vi "灰度化 (子VI).vi"(8 "错误输入（无错误）":errorcluster, 11 "引用句柄输入":T1) -> (0 "错误输出":errorcluster, 2 "图像差分":T1(plugin-control), 3 "引用句柄输出":T1)   [LabVIEW 2012]
uses:
  <vilib>/vision/Image Controls.llb/IMAQ Image.ctl
  <vilib>/vision/NI_Vision_Development_Module.lvlib
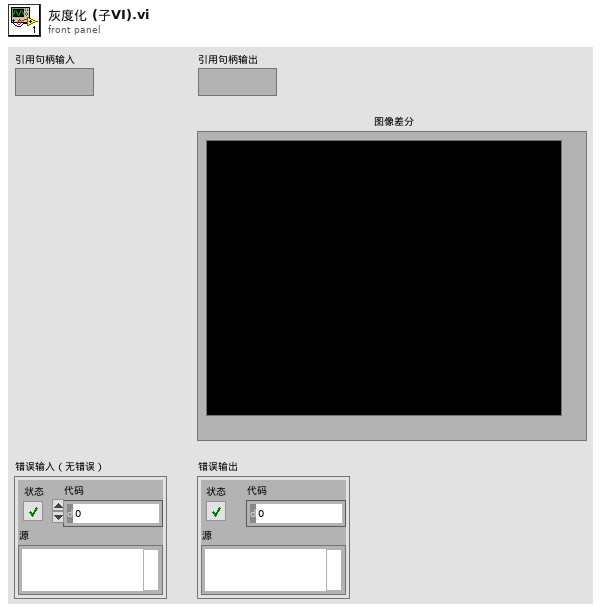
[diagram p1: front panel]
types:
  T1 = typedef "IMAQ Image.ctl" = refnum<image>
  T2 = typedef "Image Type" = u32
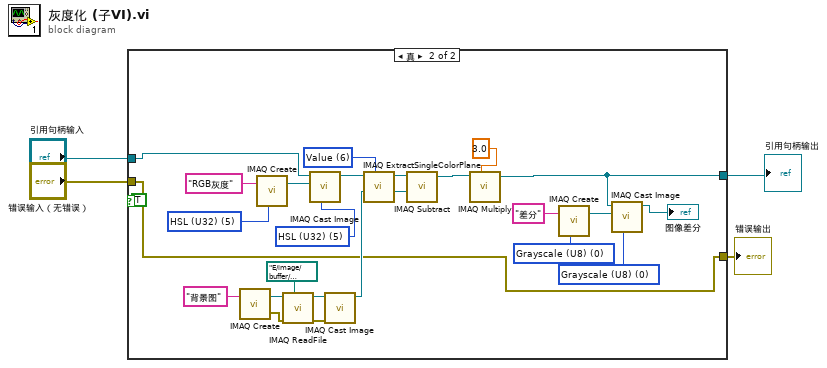
[diagram p0: block diagram]
diagram:
  n1 = case shown="真" TRUE {
    tunnel: "引用句柄输入" -> [w7 w13]
    tunnel: [w7 w12] -> w2
    tunnel: "错误输入（无错误）" -> [w6 w8]
    tunnel: [w6 w8] -> w5
    frame False {
    }
    frame True {
      w16 = T2 0 items=["Grayscale (U8)", "Grayscale (I16)", "Grayscale (SGL)", "Complex (CSG)", "RGB (U32)", "HSL (U32)", "RGB (U64)", "Grayscale (U16)"] ("Image Type")
      w18 = T2 0 items=["Grayscale (U8)", "Grayscale (I16)", "Grayscale (SGL)", "Complex (CSG)", "RGB (U32)", "HSL (U32)", "RGB (U64)", "Grayscale (U16)"] ("Image Type")
      w15 = T2 5 items=["Grayscale (U8)", "Grayscale (I16)", "Grayscale (SGL)", "Complex (CSG)", "RGB (U32)", "HSL (U32)", "RGB (U64)", "Grayscale (U16)"] ("Image Type")
      w28 = 6 items=["Red", "Green", "Blue", "Hue", "Saturation", "Luminance", "Value", "Intensity"] ("Color Plane")
      w30 = T2 5 items=["Grayscale (U8)", "Grayscale (I16)", "Grayscale (SGL)", "Complex (CSG)", "RGB (U32)", "HSL (U32)", "RGB (U64)", "Grayscale (U16)"] ("Image Type")
      n2 = call "IMAQ Create"("Image Name"="背景图") -> ("New Image"=w26:T1, "error out"=w10:errorcluster)  [unwired: 4 in]
      n3 = call "IMAQ Create"("Image Name"="RGB灰度", "Image Type"=w30) -> ("New Image"=w29:T1)  [unwired: 3 in, 1 out]
      n4 = call "IMAQ ReadFile"("File Path"=path "E:/image/buffer/background_buffer.jpg" ("背景图"), "error in (no error)"=w10, "Image"=w26) -> ("error out"=w9:errorcluster, "Image Out"=w24:T1)  [unwired: 4 in, 3 out]
      n5 = call "IMAQ Cast Image"("Image Type"=w15, "Image Dst"=w29, "Image Src"=w13) -> ("Image Dst Out"=w27:T1)  [unwired: 7 in, 1 out]
      n6 = call "IMAQ Cast Image"("error in (no error)"=w9, "Image Src"=w24) -> ("Image Dst Out"=w22:T1)  [unwired: 8 in, 1 out]
      n7 = call "IMAQ ExtractSingleColorPlane"("Color Plane"=w28, "Image Src"=w27) -> ("Image Dst Out"=w23:T1)  [unwired: 8 in, 1 out]
      n8 = call "IMAQ Subtract"("Image Src A"=w23, "Image Src B"=w22) -> ("Image Dst Out"=w21:T1)  [unwired: 5 in, 1 out]
      n9 = call "IMAQ Multiply"("Image Src A"=w21, "Constant"=sgl 3.0) -> ("Image Dst Out"=w12:T1)  [unwired: 5 in, 1 out]
      n10 = call "IMAQ Create"("Image Name"="差分", "Image Type"=w18) -> ("New Image"=w17:T1)  [unwired: 3 in, 1 out]
      n11 = call "IMAQ Cast Image"("Image Type"=w16, "Image Dst"=w17, "Image Src"=w12) -> ("Image Dst Out"=→"图像差分":T1)  [unwired: 7 in, 1 out]
    }
  }
  "错误输出" <- w5
  "引用句柄输出" <- w2
